vi "find quadratic maximum 5 points.vi"(10 "input valid":bool, 11 "xc buffer":u32[](array[numeric])=[0, 0, 0, 0, 0]) -> (2 "output valid":bool, 3 "maximum location":fxp<+/-,8,3> format="%.6g")   [LabVIEW 2010]
uses:
  <vilib>/rvi/FXPMathLib/FxpDiv/XNode/nifxpmath_Div.xnode
  <vilib>/rvi/FXPMathLib/FxpDiv/subVIs/nifxpmath_Div_SimConfig.ctl
  <vilib>/rvi/FXPMathLib/FxpDiv/simVIs/DllFxpDivTemp_sub.vi
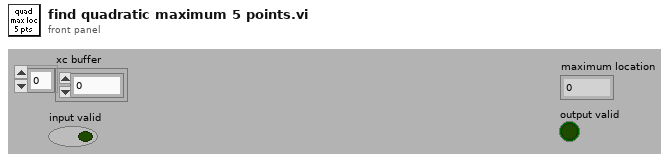
[diagram p1: front panel]
types:
  T1 = cluster{"[0]":i32, "[1]":i32, "[2]":i32, "[3]":i32, "[4]":i32}
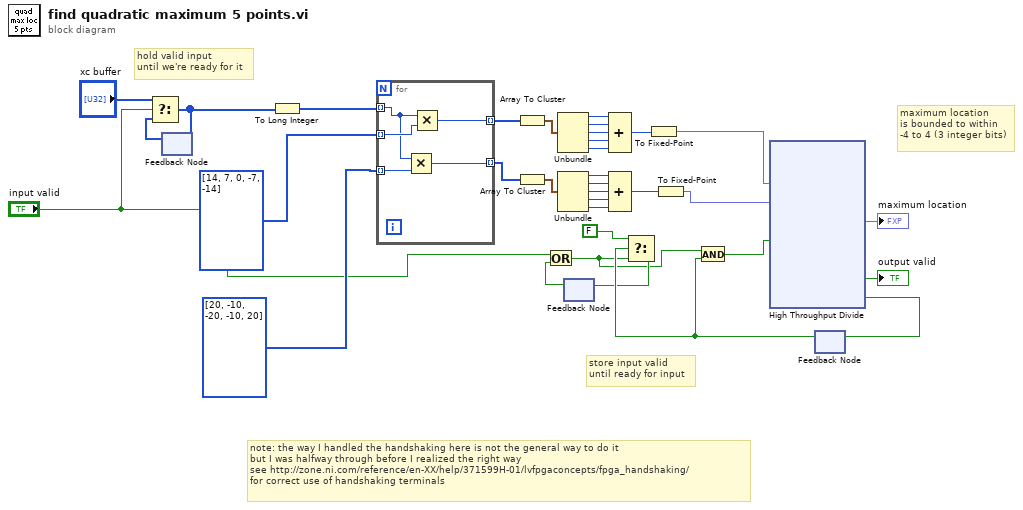
[diagram p0: block diagram]
diagram:
  # "note: the way I handled the handshaking here is not the general way to do it\nbut I was halfway through before I realized the right way\nsee http://zone.ni.com/reference/en-XX/help/371599H-01/lvfpgaconcepts/fpga_handshaking/\nfor correct use of handshaking terminals"
  # "store input valid\nuntil ready for input"
  # "hold valid input\nuntil we're ready for it"
  # "maximum location\nis bounded to within\n-4 to 4 (3 integer bits)"
  n1 = feedback #1() -> (w8:u32[])  [unwired: 1 in]
  n2 = Select(t="xc buffer", s="input valid", f=w8) -> (s? t:f=w7:u32[])
  n3 = feedback-in #1(w7) -> ()
  n4 = To Long Integer(number=w7) -> (32bit integer=w28:i32[])
  n5 = for {
    tunnel: w28 -> [w36] mode=indexing
    tunnel: i32[] [14, 7, 0, -7, -14] ("xc buffer") -> [w39] mode=indexing
    tunnel: i32[] [20, -10, -20, -10, 20] ("xc buffer") -> [w37] mode=indexing
    tunnel: [w38] -> w27 mode=indexing
    tunnel: [w35] -> w14 mode=indexing
    n6 = Multiply(x=w36, y=w37) -> (x*y=w35:i32)
    n7 = Multiply(x=w36, y=w39) -> (x*y=w38:i32)
  }
  n8 = Array To Cluster(array=w27) -> (cluster=w26:T1)
  n9 = Array To Cluster(array=w14) -> (cluster=w20:T1)
  n10 = Unbundle(w26) -> ("[0]"=w25:i32, "[1]"=w24:i32, "[2]"=w23:i32, "[3]"=w22:i32, "[4]"=w21:i32)
  n11 = Unbundle(w20) -> ("[0]"=w19:i32, "[1]"=w18:i32, "[2]"=w17:i32, "[3]"=w16:i32, "[4]"=w15:i32)
  n12 = feedback #2() -> (w4:bool)  [unwired: 1 in]
  n13 = Or(x="input valid", y=w4) -> (x .or. y?=w2:bool)
  n14 = Compound Arithmetic op=ADD(w25, w24, w23, w22, w21) -> (w13:i32)
  n15 = Compound Arithmetic op=ADD(w19, w18, w17, w16, w15) -> (w12:i32)
  n16 = To Fixed-Point(number=w13) -> (fixed-point=w11:fxp<+/-,20,20>)  [unwired: 1 in]
  n17 = To Fixed-Point(number=w12) -> (fixed-point=w10:fxp<+/-,20,20>)  [unwired: 1 in]
  n18 = feedback #3() -> (w6:bool)  [unwired: 1 in]
  n19 = Select(t=FALSE, s=w6, f=w2) -> (s? t:f=w3:bool)
  n20 = feedback-in #2(w3) -> ()
  n21 = And(x=w2, y=w6) -> (x .and. y?=w9:bool)
  n22 = xnode "High Throughput Divide"("x"=w11, "y"=w10, "input valid"=w9) -> ("x/y"=→"maximum location":fxp<+/-,8,3>, "output valid"=→"output valid":bool, "ready for input"=w34:bool)  [unwired: 1 in]
  n23 = feedback-in #3(w34) -> ()
